vi "Error__slk_mt.vi"(8 "error":enum16{"No This Frame Name"}(ring)) -> (0 "error out":errorcluster)   [LabVIEW 2010, in "Lazyboots Menu Tool.lvlib" / "CaseModel__slk_mt.lvclass"]
uses:
  CaseModel__slk_mt.lvclass
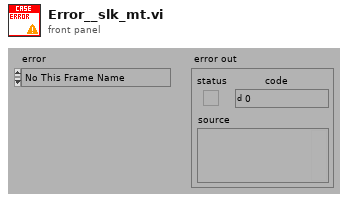
[diagram p1: front panel]
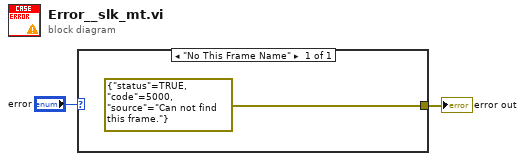
[diagram p0: block diagram]
diagram:
  n1 = case shown="\"No This Frame Name\"" "error" {
    tunnel: [errorcluster {"status"=TRUE, "code"=5000, "source"="Can not find this frame."} ("error out")] -> w1
    frame "No This Frame Name" {
    }
  }
  "error out" <- w1
